vi "Set Values.vi"(8 "error in (no error)":errorcluster, 9 "Duration":dbl, 10 "Target":dbl, 11 "Rate Step in":refnum<class "Rate Duration.lvclass">) -> (0 "error out":errorcluster, 3 "Rate Step out":refnum<class "Rate Duration.lvclass">)   [LabVIEW 2018, in "Temp Recipe.lvlib" / "Rate Duration.lvclass"]
uses:
  Rate Duration.lvclass
  C:/dev/source/Systems/NI Week/Temperature Recipe/Temp Recipe/Recipe Step/Recipe Step.lvclass
  Rate Duration.lvclass/Rate Duration.ctl
  Recipe Step/Recipe Step.lvclass
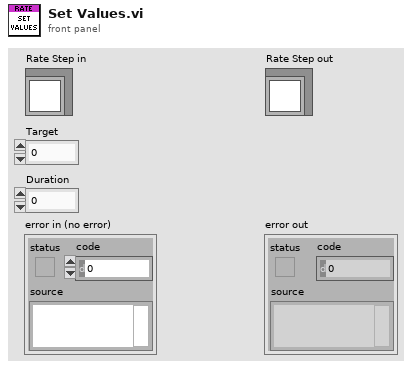
[diagram p1: front panel]
types:
  T1 = typedef "Temp Recipe.lvlib/Rate Duration.lvclass/Ref Data.ctl" = cluster{"Target":dbl, "Duration":dbl}
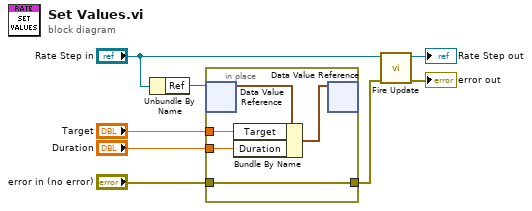
[diagram p0: block diagram]
diagram:
  n1 = Unbundle By Name("Rate Step in") -> ("Ref"=w8:refnum<data-value>)
  n2 = in-place {
    in-place-border: "Target" -> [w11]
    in-place-border: "Duration" -> [w10]
    in-place-border: "error in (no error)" -> [w9]
    in-place-border: [w9] -> w3
    n3 = in-place-dvr #1(w8) -> (w13:T1)  [unwired: 1 out]
    n4 = Bundle By Name(cluster=w13, "Target"=w11, "Duration"=w10) -> (w12:T1)
    n5 = in-place-dvr #1(w12) -> ()  [unwired: 2 out]
  }
  n6 = call "Fire Update.vi"("error in (no error)"=w3, "Recipe Step in"="Rate Step in") -> ("error out"=→"error out":errorcluster, "Recipe Step out"=→"Rate Step out":refnum<class "Rate Duration.lvclass">)  [unwired: 8 in]
